vi "Robot Global Data.vi"() -> ()   [LabVIEW 2016]
doc: "This global VI can contain as many global variables as you need. Place a control on the panel, give it a good name. To read or write to it from a VI, drag the icon to the diagram of that VI. You can also drag from the project. Click on the node to change which global you access. You shouldn't have multiple locations writing to a global or it will cause a race-condition."
uses:
  <vilib>/Rock Robotics/WPI/Camera/WPI_CameraImageSize.ctl
  <vilib>/Rock Robotics/WPI/DriverStation/WPI_DriverStationRobotMode2.ctl
  <vilib>/Rock Robotics/WPI/Gyro/WPI_GyroDevRef.ctl
  <vilib>/Rock Robotics/SystemInterfaces/AI/FPGA_AIChannel.ctl
  <vilib>/Rock Robotics/SystemInterfaces/spilib/spi_bus.ctl
  <vilib>/Rock Robotics/WPI/Accelerometer/WPI_AccelerometerDevRef.ctl
  <vilib>/Rock Robotics/WPI/Accelerometer/WPI_AccelerometerScaling.ctl
  <vilib>/Rock Robotics/WPI/Accelerometer/WPI_AccelerometerAnalogChannels.ctl
  <vilib>/Rock Robotics/SystemInterfaces/i2clib/i2c_bus.ctl
  <vilib>/Rock Robotics/WPI/Accelerometer/ADXL345 Range.ctl
  <vilib>/Rock Robotics/WPI/Accelerometer/WPI_AccelerometerADXL345 Axes.ctl
  <vilib>/Rock Robotics/WPI/MotorControl/WPI_MotorControlDeviceRef.ctl
  <vilib>/Rock Robotics/WPI/MotorControl/WPI_MotorControlType.ctl
  <vilib>/Rock Robotics/SystemInterfaces/DIO/FPGA_DIOPWMChannel.ctl
  <vilib>/Rock Robotics/WPI/PWM/WPI_PWMDeadband.ctl
  HopperStates.ctl
panel:
  out "Toggle Reverse Variable 2":dbl
  out "Shooter Speed":dbl
  out "Shooter Reverse":bool
  out "Shooter Preset":bool
  out "Pickup":bool
  out "Preset":bool
  out "Agitator":bool
  out "US Average":dbl
  out "Center X Offset":i32
  in  "StatesForHopper":T1
  in  "changeState":T1
  in  "currentState":T1
  out "Gear Flip Servo":bool
  in  "Auto Selector":i32
  out "Fast Mode":bool
  out "Results":T2 {"Score" format="%#_3g"; "Pixels"."Rectangle"."Numeric 5" format="%#_3g"; "Pixels"."Rectangle"."Numeric 3" format="%#_3g"; "Pixels"."Rectangle"."Numeric 2" format="%#_3g"; "Pixels"."Rectangle"."Numeric" format="%#_3g"; "Normalized"."Rectangle"."Numeric 5" format="%#_2g"; "Normalized"."Rectangle"."Numeric 3" format="%#_2g"; "Normalized"."Rectangle"."Numeric 2" format="%#_2g"; "Normalized"."Rectangle"."Numeric" format="%#_2g"; "Normalized"."Center"."?" format="%#_3g"; "Normalized"."Center"."?" format="%#_3g"; "Distance (ft)" format="%#_3g"}
  out "Tick Count(Ticks) 2":u32 caption="Tick Count(Ticks) 1"
  out "Tick Count(Ticks)":u32 caption="Tick Count(Ticks) 2"
  out "Alligned":bool
  in  "image size Cam 2":T3
  out "Battery Voltage Array":dbl[](array[numeric])
  out "Teleop State":T4(ring)
  out "Button 1":bool
  out "Button 3":bool
  out "Button 2":bool
  out "Button 4":bool
  out "Tick Count(mSec)":u32
  out "Change Profile":bool
  out "Manual Lower Hopper":bool
  out "Manual Raise Hopper":bool
  out "Distance Moved (Feet)":dbl
  out "Encoder Auto":bool
  out "Gear is Present (Photoeye)":bool
  out "Encoder Index Pin State":bool
  out "Encoder B Pin State":bool
  out "Encoder A Pin State":bool
  out "Encoder Index Count":dbl
  out "Encoder Velocity":dbl
  out "Encoder Position":dbl
  out "US Raw Difference":dbl
  out "Ball Dump Servo Up/Down":bool
  out "Ball Dump Servo (Down)":dbl
  out "Ball Dump Servo (Up)":dbl
  out "Backboard Right Up Position":dbl
  out "Backboard Left Up Position":dbl
  out "Backboard Left Down":bool
  out "Backboard Right Down":bool
  out "US Sweeper Equality":dbl
  out "US Sweeper (Raw) Right":dbl
  out "US Sweeper (Raw) Left":dbl
  out "US Sweeper Left":dbl
  out "US Sweeper Right":dbl
  out "Min Talon bat Voltage":dbl
  out "Max DT current":dbl
  out "DT Talon Ref Array":T5[](array[typedef])
  out "INAV OK":bool
  out "INAV Sensor Cluster":T18 {"GyroDevRef"."Sample Rate" min=0.25 max=100.0 step=0.25; "AccelerometerDevRef"."Device Address" format="%.0x"; "AccelerometerDevRef"."Accel Range" items=["+/- 2 g", "+/- 4 g", "+/- 8 g", "+/- 16 g"]}
  out "VComp Enable":bool
  out "Toggle Reverse Variable":dbl
  out "Photoeye - Back Down":bool
  out "Photoeye - Back Up":bool
  out "Photoeye - Front Down":bool
  out "Photoeye - Front Up":bool
  out "Backboard (Left) Down Position":dbl
  out "Backboard Left Up":bool
  out "Backboard Right Up":bool
  out "Backboard (Right) Down Position":dbl
  out "Percise Slow Mode":bool
  out "Comparison (=)":bool
  out "Comparison Output (>=)":bool
  out "Comparison Output (<=)":bool
  out "Comparison Output":dbl
  out "US Raw Left":dbl
  out "US Raw Right":dbl
  out "Nominal Status (Reverse)":dbl
  out "Nominal Status (Forward)":dbl
  out "Auto Allignment":bool
  out "US Equality":dbl
  out "US Gear Left (-)":dbl
  out "US Gear Right (+)":dbl
  out "Limit Switch - Peg Hit Web of Gear (Indicator)":bool
  out "Limit Switch - Peg through Gear (Indicator)":bool
  out "Limit Switch - Gear is Present (Indicator)":bool
  out "Lift Motor - Reverse":bool
  out "Stop Lift Motor":bool
  out "Initiate Lift Motor + System":bool
  out "Ball Intake Motor - Reverse":bool
  out "Toggle - On/Off - Intake and Ball Elevator Motors":bool
  out "Manual - Rear Cloth Roller (Down)":bool
  out "Manual - Rear Cloth Roller (Up)":bool
  out "Manual - Front Cloth Roller (Down)":bool
  out "Manual - Front Cloth Roller (Up)":bool
  out "Manual - Wall to Boiler (Down)":bool
  out "Manual - Wall to Boiler (Up)":bool
  out "Activate Ball Dump":bool
  out "Drop Rear Gear Wall":bool
  out "Manual - Rear Gear Wall (Down)":bool
  out "Manual - Rear Gear Wall (Up)":bool
  out "Indicator - Gear Loaded + Drop Wall":bool
  out "Activate Lift Camera":bool
  out "Autonomous Gear Actuation":bool
  out "Activate Wall Alignment":bool
  out "Drive (Rear - Forward Toggle)":bool
  in  "Camera Exposure":dbl
  out "Slow Mode":bool
  in  "Robot Mode":T19
  in  "image size":T3
  in  "Enable Vision":bool
  # "Drive System Buttons"
  # "Gear System Buttons/Indicators"
  # "__________________________________________________________________________________________________________"
  # "---"
  # "---"
  # "---"
  # "______________________________"
  # "---"
  # "---"
  # "---"
  # "---"
  # "______________________________________________"
  # "___________________________________________________"
  # "Ball System"
  # "Rope System"
  # "---"
  # "Autonomous"
  # "---"
  # "---"
  # "---"
  # "---"
  # "---"
  # "---"
  # "---"
  # "---"
  # "____________________________________________________________________________________________"
  # "Analog"
  # "XRS"
  # "ADXL"
  # "Analog"
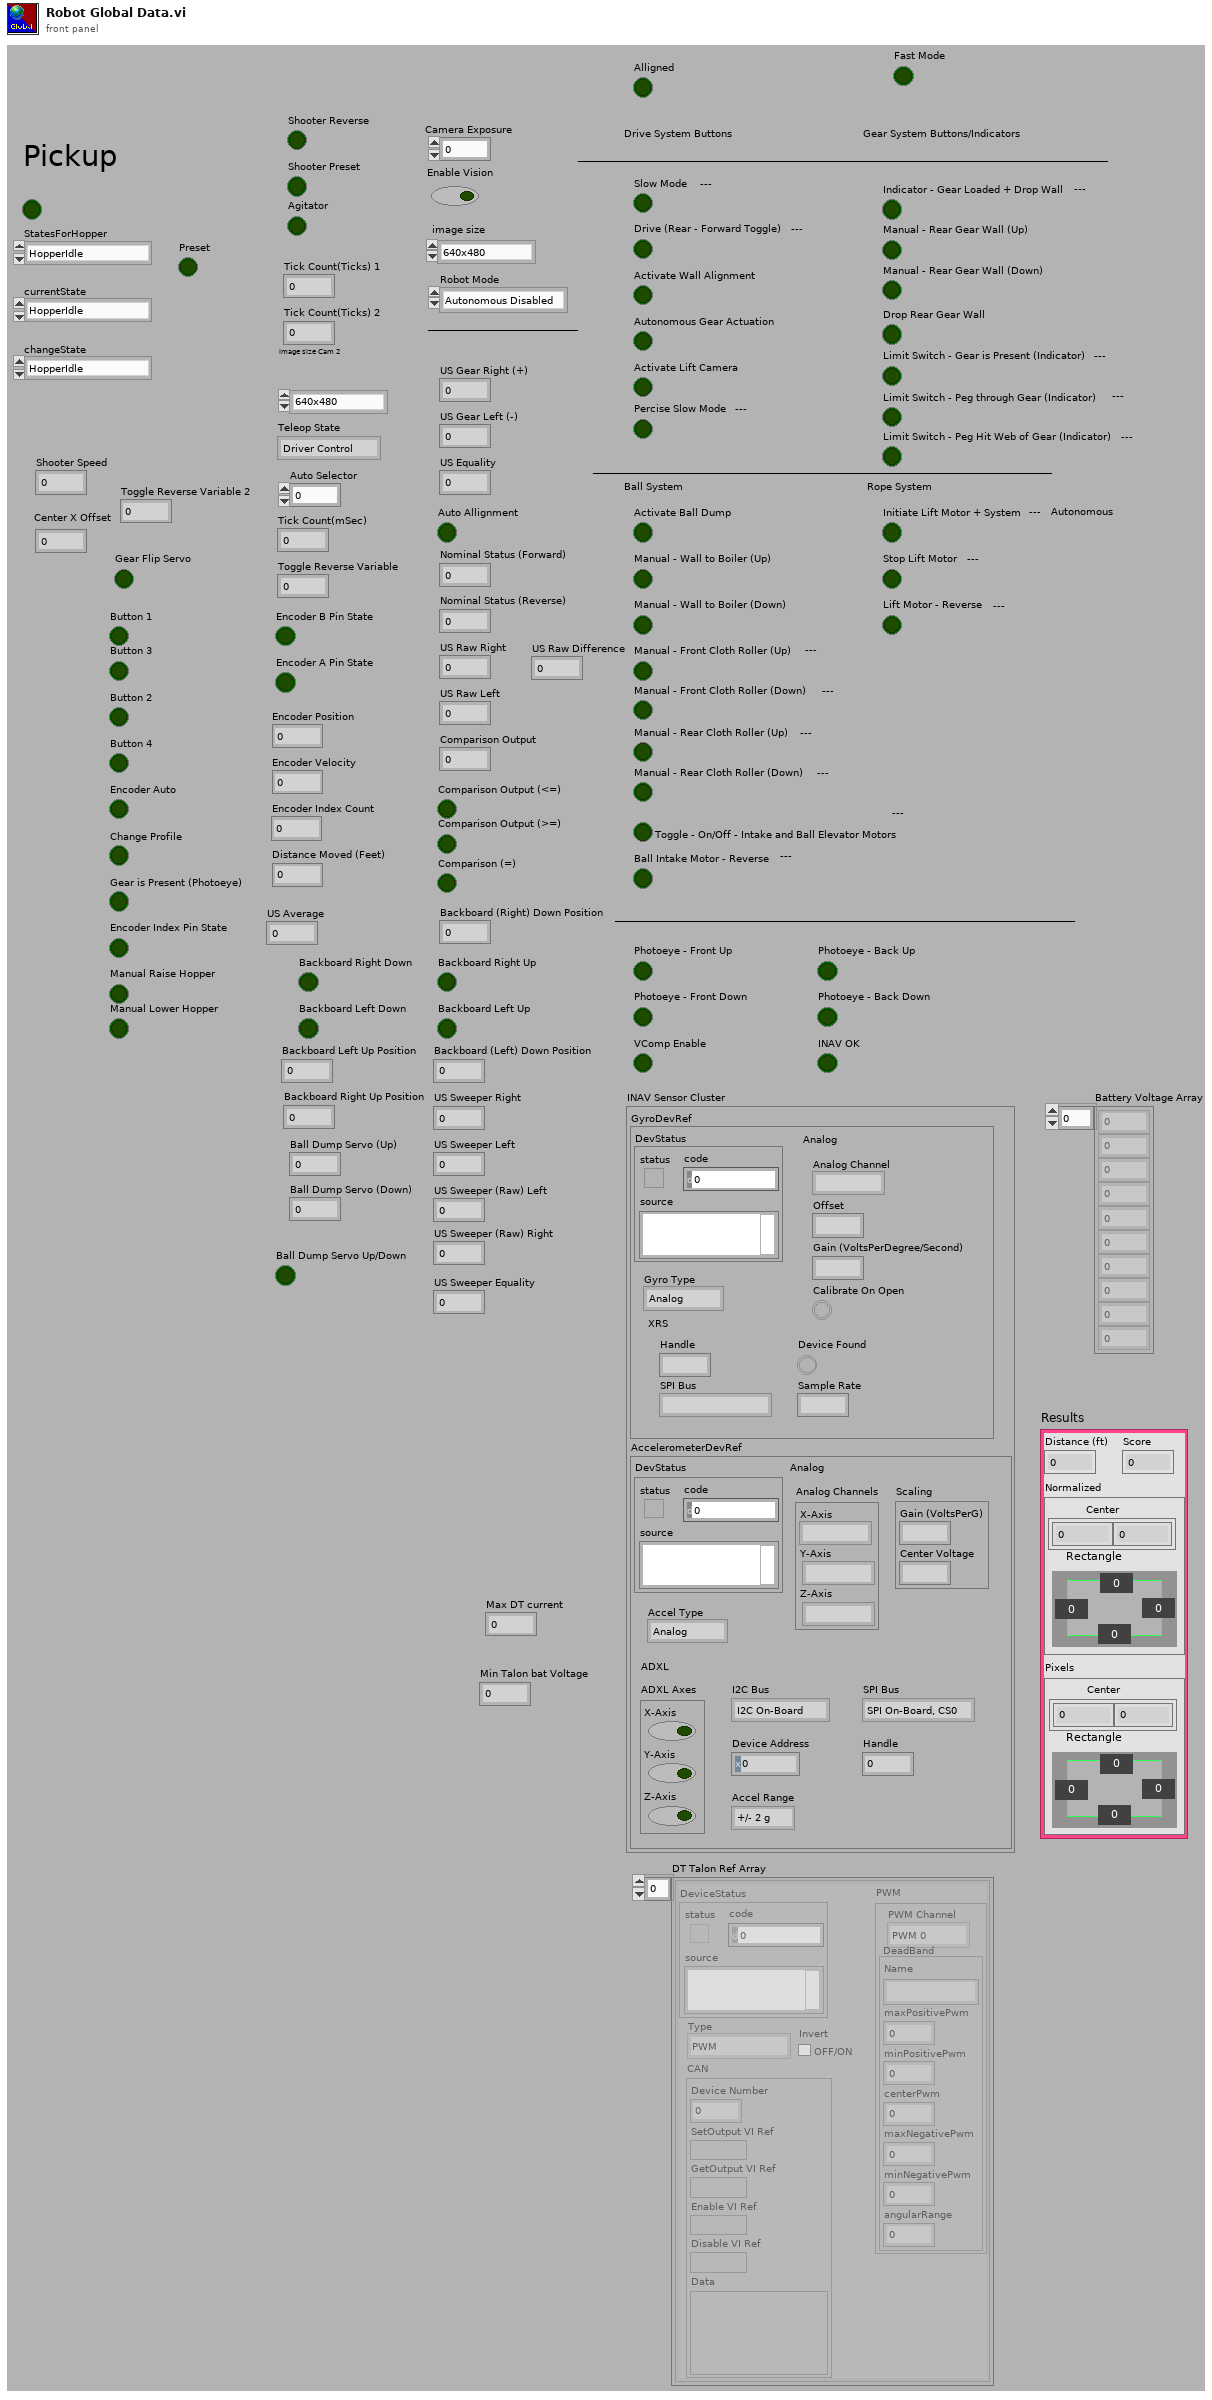
[diagram p1: front panel]
types:
  T1 = typedef "HopperStates.ctl" = enum16{"HopperIdle", "ManualRaiseHopper", "ManualLowerHopper", "AutoRaiseHopper", "AutoLowerHopper", "AtTop", "AtBottom"}
  T2 = cluster{"Distance (ft)":dbl, "Score":dbl, "Normalized":cluster{"Center":cluster{dbl, dbl}, "Rectangle":cluster{"Numeric":dbl, "Numeric 2":dbl, "Numeric 3":dbl, "Numeric 5":dbl}}, "Pixels":cluster{"Center":cluster{dbl, dbl}, "Rectangle":cluster{"Numeric":dbl, "Numeric 2":dbl, "Numeric 3":dbl, "Numeric 5":dbl}}}
  T3 = typedef "WPI_CameraImageSize.ctl" = enum16{"640x480", "320x240", "160x120", "Custom"}
  T4 = enum16{"Driver Control", "Gear Coarse Adjust", "Gear Fine Adjust"}
  T5 = typedef "WPI_MotorControlDeviceRef.ctl" = cluster{"DeviceStatus":errorcluster, "Type":T6, "PWM":cluster{"PWM Channel":T7, "DeadBand":T8}, "CAN":cluster{"Device Number":u8, "SetOutput VI Ref":variant, "GetOutput VI Ref":variant, "Enable VI Ref":variant, "Disable VI Ref":variant, "Data":variant}, "Invert":bool}
  T6 = typedef "WPI_MotorControlType.ctl" = enum16{"PWM", "CAN"}
  T7 = typedef "FPGA_DIOPWMChannel.ctl" = enum8{"PWM 0", "PWM 1", "PWM 2", "PWM 3", "PWM 4", "PWM 5", "PWM 6", "PWM 7", "PWM 8", "PWM 9", "PWM MXP 0", "PWM MXP 1", "PWM MXP 2", "PWM MXP 3", "PWM MXP 4", "PWM MXP 5", "PWM MXP 6", "PWM MXP 7", "PWM MXP 8", "PWM MXP 9", "Invalid"}
  T8 = typedef "WPI_PWMDeadband.ctl" = cluster{"Name":string, "maxPositivePwm":i32, "minPositivePwm":i32, "centerPwm":i32, "maxNegativePwm":i32, "minNegativePwm":i32, "angularRange":u16}
  T9 = typedef "WPI_GyroDevRef.ctl" = cluster{"DevStatus":errorcluster, "Analog Channel":T10, "Offset":dbl, "Gain (VoltsPerDegree/Second)":dbl, "Gyro Type":enum16{"Analog", "XRS450"}, "Handle":i32, "SPI Bus":T11, "Device Found":bool, "Sample Rate":dbl, "Calibrate On Open":bool}
  T10 = typedef "FPGA_AIChannel.ctl" = enum8{"AI 0", "AI 1", "AI 2", "AI 3", "AI MXP 0", "AI MXP 1", "AI MXP 2", "AI MXP 3", "Invalid"}
  T11 = typedef "spi_bus.ctl" = enum16{"SPI On-Board, CS0", "SPI On-Board, CS1", "SPI On-Board, CS2", "SPI On-Board, CS3", "SPI MXP", "Invalid"}
  T12 = typedef "WPI_AccelerometerDevRef.ctl" = cluster{"DevStatus":errorcluster, "Scaling":T13, "Analog Channels":T14, "I2C Bus":T15, "SPI Bus":T11, "Accel Range":T16, "ADXL Axes":T17, "Handle":i32, "Device Address":u8, "Accel Type":enum16{"Analog", "ADXL345 I2C", "ADXL345 SPI", "Internal", "ADXL362 SPI"}}
  T13 = typedef "WPI_AccelerometerScaling.ctl" = cluster{"Gain (VoltsPerG)":dbl, "Center Voltage":dbl}
  T14 = typedef "WPI_AccelerometerAnalogChannels.ctl" = cluster{"X-Axis":T10, "Y-Axis":T10, "Z-Axis":T10}
  T15 = typedef "i2c_bus.ctl" = enum16{"I2C On-Board", "I2C MXP", "Invalid"}
  T16 = typedef "ADXL345 Range.ctl" = u8
  T17 = typedef "WPI_AccelerometerADXL345 Axes.ctl" = cluster{"X-Axis":bool, "Y-Axis":bool, "Z-Axis":bool}
  T18 = cluster{"GyroDevRef":T9, "AccelerometerDevRef":T12}
  T19 = typedef "WPI_DriverStationRobotMode2.ctl" = enum16{"Autonomous Disabled", "Autonomous Enabled", "Teleop Disabled", "Teleop Enabled", "Disconnected", "Finish", "Test Disabled", "Test Enabled", "Emergency Stopped"}
diagram:
